vi "SortActions.vi"(11 "rule in":T1) -> (3 "rule out":T1)   [LabVIEW 2017, in "TrendAlarm.lvlib"]
uses:
  <vilib>/addons/InsightCM/Devices/Shared/Common/TrendAlarm/TrendAlarm.lvlib
  <vilib>/addons/InsightCM/MessageBus/Base/controls/TrendAlarmRule.ctl
  <vilib>/addons/InsightCM/MessageBus/Base/controls/TrendAlarmLevel.ctl
  <vilib>/addons/InsightCM/MessageBus/Base/controls/AlarmAction.ctl
  <vilib>/addons/InsightCM/MessageBus/Base/controls/KeyValuePair.ctl
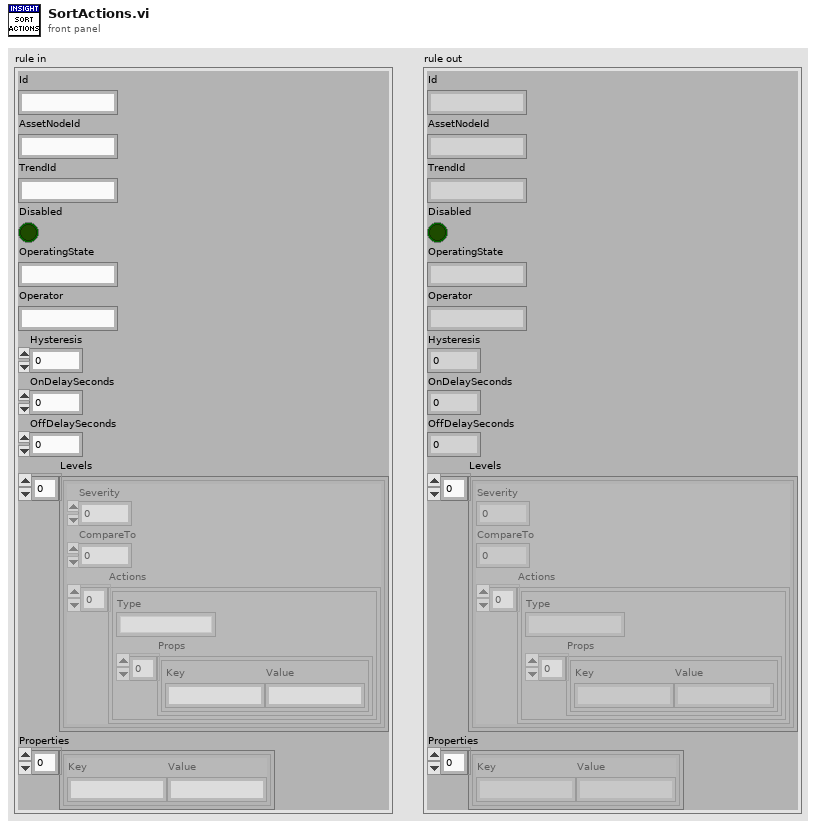
[diagram p1: front panel]
types:
  T1 = typedef "TrendAlarmRule.ctl" = cluster{"Id":string, "AssetNodeId":string, "TrendId":string, "Disabled":bool, "OperatingState":string, "Operator":string, "Hysteresis":dbl, "OnDelaySeconds":dbl, "OffDelaySeconds":dbl, "Levels":T2[], "Properties":T4[]}
  T2 = typedef "TrendAlarmLevel.ctl" = cluster{"Severity":i32, "CompareTo":dbl, "Actions":T3[]}
  T3 = typedef "AlarmAction.ctl" = cluster{"Type":string, "Props":T4[]}
  T4 = typedef "KeyValuePair.ctl" = cluster{"Key":string, "Value":string}
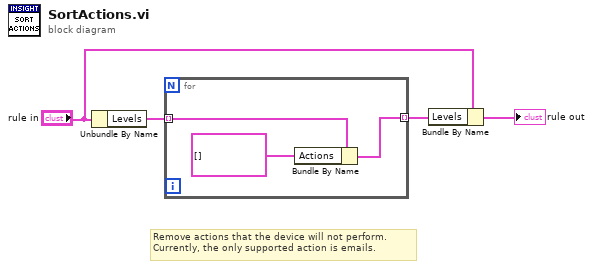
[diagram p0: block diagram]
diagram:
  # "Remove actions that the device will not perform.  \nCurrently, the only supported action is emails."
  n1 = Unbundle By Name("rule in") -> ("Levels"=w4:T2[])
  n2 = for {
    tunnel: w4 -> [w7] mode=indexing
    tunnel: [w5] -> w2 mode=indexing
    n3 = Bundle By Name(cluster=w7, "Actions"=T3[] []) -> (w5:T2)
  }
  n4 = Bundle By Name(cluster="rule in", "Levels"=w2) -> (→"rule out":T1)
